vi "Convert Database Data to List.vi"(8 "error in (no error)":errorcluster, 10 "FetchedData":variant[](array[variant]), 11 "NormalQDFunc in":refnum<class "QDDialogList.lvclass">) -> (0 "error out":errorcluster, 1 "QDFunction Acronym":string, 2 "QDFunction Name":string, 3 "NormalQDFunc out":refnum<class "QDDialogList.lvclass">)   [LabVIEW 2015, in "QDDialogList.lvclass"]
uses:
  QDDialogList.lvclass
  QDDialogList.lvclass/QDDialogList.ctl
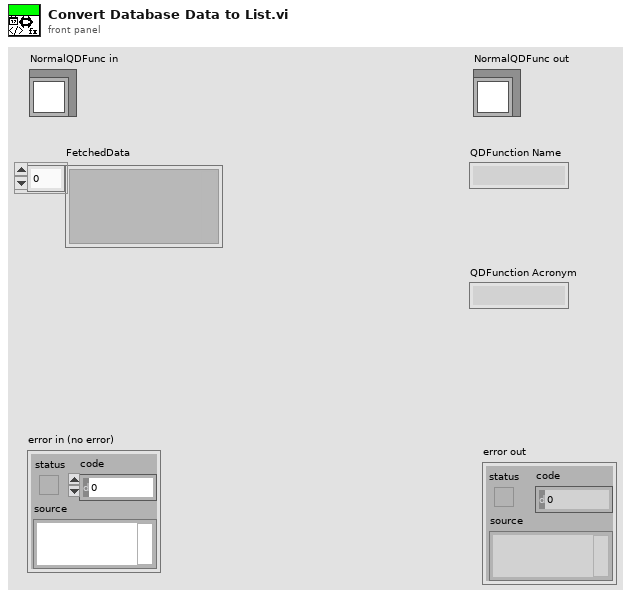
[diagram p1: front panel]
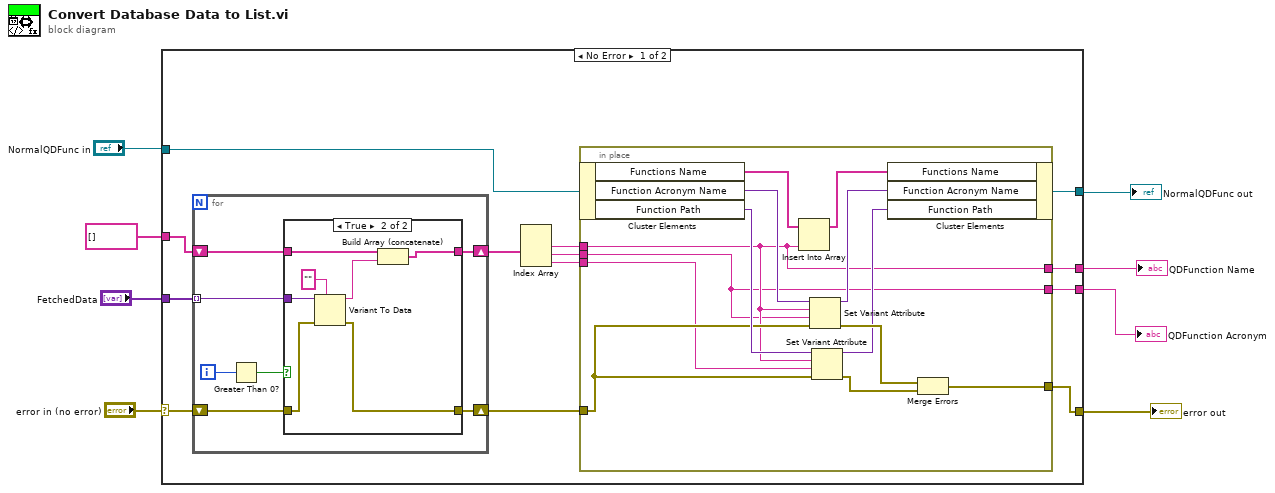
[diagram p0: block diagram]
diagram:
  n1 = case shown="No Error" "error in (no error)" {
    selector: "error in (no error)" -> [w20 w52]
    tunnel: "FetchedData" -> [w21 _]
    tunnel: string[] [] -> [w19 _]
    tunnel: [w11 w52] -> w5
    tunnel: "NormalQDFunc in" -> [w17 w51]
    tunnel: [w13 w51] -> w3
    tunnel: [w10 _] -> w2
    tunnel: [w9 _] -> w1
    frame No Error {
      n2 = for {
        tunnel: w21 -> [w39] mode=indexing
        shift-right: [w36] -> w12
        shift-left: w20 -> [w38]
        shift-right: [w35] -> w18
        shift-left: w19 -> [w37]
        i -> [w41]
        n3 = Greater Than 0?(x=w41) -> (x > 0?=w40:bool)
        n4 = case shown="True" w40 {
          tunnel: w39 -> [_ w50]
          tunnel: w38 -> [w42 w48]
          tunnel: w37 -> [w43 w47]
          tunnel: [w42 w45] -> w36
          tunnel: [w43 w44] -> w35
          frame False {
          }
          frame True {
            n5 = Variant To Data(error in=w48, type="", Variant=w50) -> (data=w46:string, error out=w45:errorcluster)
            n6 = Build Array (concatenate)(w47, w46) -> (w44:string[])
          }
        }
      }
      n7 = Index Array(array=w18) -> (element #1=w16:string, element #2=w15:string, element #3=w14:string)  [unwired: 3 in]
      n8 = in-place {
        in-place-border: w16 -> [w24]
        in-place-border: w15 -> [w22]
        in-place-border: w14 -> [w23]
        in-place-border: w12 -> [w29]
        in-place-border: [w26] -> w11
        in-place-border: [w24] -> w10
        in-place-border: [w22] -> w9
        n9 = in-place-cluster #1(w17) -> ("Functions Name"=w34:string[], "Function Acronym Name"=w32:variant, "Function Path"=w30:variant)
        n10 = Insert Into Array(array=w34, new element=w24) -> (w33:string[])  [unwired: 1 in]
        n11 = Set Variant Attribute(Variant=w32, name=w24, value=w22, error in=w29) -> (Variant out=w31:variant, error out=w28:errorcluster)  [unwired: 1 out]
        n12 = Set Variant Attribute(Variant=w30, name=w24, value=w23, error in=w29) -> (Variant out=w25:variant, error out=w27:errorcluster)  [unwired: 1 out]
        n13 = in-place-cluster #1("Functions Name"=w33, "Function Acronym Name"=w31, "Function Path"=w25) -> (w13:refnum<class "QDDialogList.lvclass">)
        n14 = Merge Errors(w28, w27) -> (w26:errorcluster)
      }
    }
    frame Error {
    }
  }
  "error out" <- w5
  "NormalQDFunc out" <- w3
  "QDFunction Name" <- w2
  "QDFunction Acronym" <- w1
